vi "SetupNotifyer.vi"(8 "error in (no error)":errorcluster, 10 "Status Notifier":refnum<notifier>, 11 "Microscope_RM21 in":refnum<class "Microscope_RM21.lvclass">) -> (0 "error out":errorcluster, 3 "Microscope_RM21 out":refnum<class "Microscope_RM21.lvclass">)   [LabVIEW 2020, in "Microscope_RM21.lvlib" / "Microscope_RM21.lvclass"]
uses:
  Microscope_RM21.lvclass
  Microscope_RM21.lvclass/Microscope_RM21.ctl
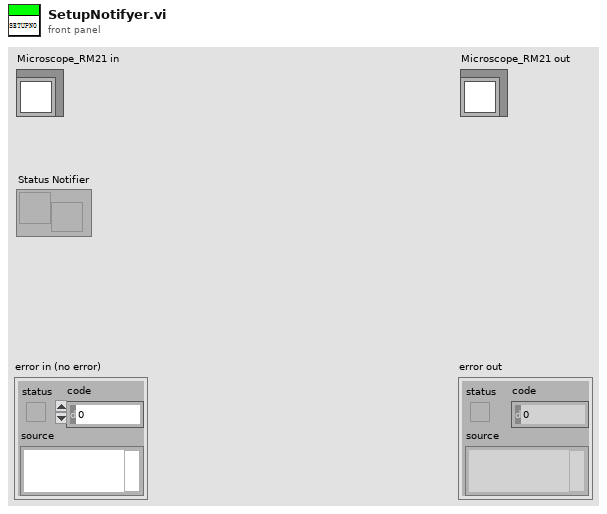
[diagram p1: front panel]
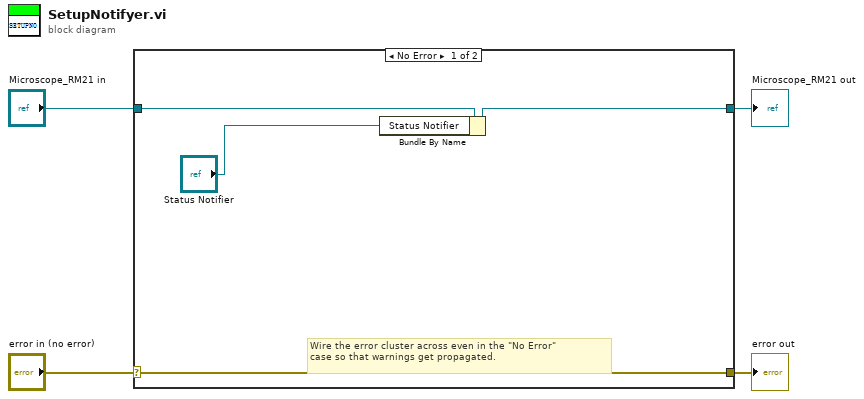
[diagram p0: block diagram]
diagram:
  n1 = case shown="No Error" "error in (no error)" {
    selector: "error in (no error)" -> [w7 w10]
    tunnel: [w7 w10] -> w3
    tunnel: [w6 w9] -> w1
    tunnel: "Microscope_RM21 in" -> [w8 w9]
    frame No Error {
      # "Wire the error cluster across even in the \"No Error\"\ncase so that warnings get propagated."
      n2 = Bundle By Name(cluster=w8, "Status Notifier"="Status Notifier") -> (w6:refnum<class "Microscope_RM21.lvclass">)
    }
    frame Error {
    }
  }
  "error out" <- w3
  "Microscope_RM21 out" <- w1
